vi "Stop Respective Module.vi"(8 "error in (no error)":errorcluster) -> (0 "error out":errorcluster)   [LabVIEW 2021, in "User Interface.lvlib"]
uses:
  User Interface.lvlib
  Database/Database.lvlib
  DAQ Hardware/DAQ Hardware.lvlib
  DAQ IO/DAQ IO.lvlib
  ARINC/ARINC.lvlib
  DC PWS/DC PWS.lvlib
  DMM/DMM.lvlib
  Func Generator/Func Generator.lvlib
  Oscilloscope/Oscilloscope.lvlib
  S-Matrix/S-Matrix.lvlib
  Environment Chamber/Environment Chamber.lvlib
  CAN/CAN.lvlib
  CVT/CVT.lvlib
  Error Log/Error Log.lvlib
  Calibration/Calibration.lvlib
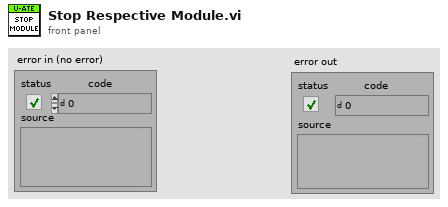
[diagram p1: front panel]
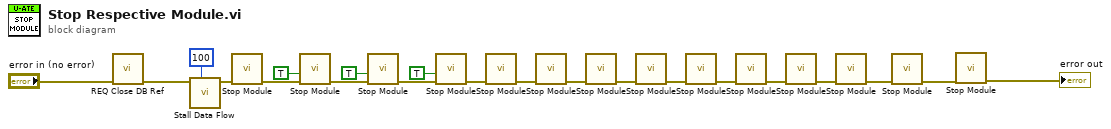
[diagram p0: block diagram]
diagram:
  n1 = call "REQ Close DB Ref.vi"("error in"="error in (no error)") -> ("error out"=w13:errorcluster)  [unwired: 10 in]
  n2 = call "Stall Data Flow.vi"("milliseconds to wait"=u32 100, "error in (no error)"=w13) -> ("error out"=w12:errorcluster)  [unwired: 9 in]
  n3 = call "Stop Module.vi"("error in"=w12) -> ("error out"=w21:errorcluster)  [unwired: 10 in]
  n4 = call "Stop Module.vi"("error in"=w21, "Wait for Module to Stop? (F)"=TRUE) -> ("error out"=w5:errorcluster)  [unwired: 9 in]
  n5 = call "Stop Module.vi"("error in"=w5, "Wait for Module to Stop? (F)"=TRUE) -> ("error out"=w17:errorcluster)  [unwired: 9 in]
  n6 = call "Stop Module.vi"("error in"=w17, "Wait for Module to Stop? (F)"=TRUE) -> ("error out"=w16:errorcluster)  [unwired: 9 in]
  n7 = call "Stop Module.vi"("error in"=w16) -> ("error out"=w18:errorcluster)  [unwired: 10 in]
  n8 = call "Stop Module.vi"("error in"=w18) -> ("error out"=w15:errorcluster)  [unwired: 10 in]
  n9 = call "Stop Module.vi"("error in"=w15) -> ("error out"=w6:errorcluster)  [unwired: 10 in]
  n10 = call "Stop Module.vi"("error in"=w6) -> ("error out"=w10:errorcluster)  [unwired: 10 in]
  n11 = call "Stop Module.vi"("error in"=w10) -> ("error out"=w9:errorcluster)  [unwired: 10 in]
  n12 = call "Stop Module.vi"("error in"=w9) -> ("error out"=w8:errorcluster)  [unwired: 10 in]
  n13 = call "Stop Module.vi"("error in"=w8) -> ("error out"=w7:errorcluster)  [unwired: 10 in]
  n14 = call "Stop Module.vi"("error in"=w7) -> ("error out"=w3:errorcluster)  [unwired: 10 in]
  n15 = call "Stop Module.vi"("error in"=w3) -> ("error out"=w2:errorcluster)  [unwired: 10 in]
  n16 = call "Stop Module.vi"("error in"=w2) -> ("error out"=→"error out":errorcluster)  [unwired: 10 in]
